vi "Call Fade-In Async.vi"(4 "Close on Fade-Out [T]":bool=TRUE, 5 "Delay (ms) [0]":i32, 6 "Fade Direction [Fade In]":enum16{"Fade In", "Fade Out"}(ring), 7 "Fade-In Time (ms)":u32=200, 8 "error in (no error)":errorcluster, 11 "Calling VI":refnum<vi>) -> (0 "error out":errorcluster)   [LabVIEW 2017]
doc: "Calls the Fade In/Out VI asynchronously so that other operations are not interrupted by this nicety.\n\nIf the calling VI Ref is not wired, the calling VIs parent is assumed, which is usally what you want."
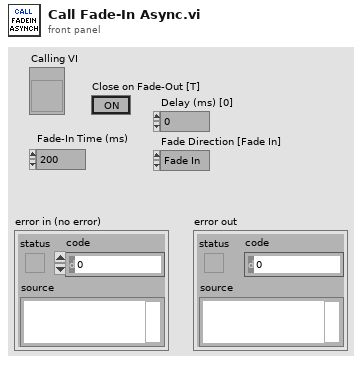
[diagram p1: front panel]
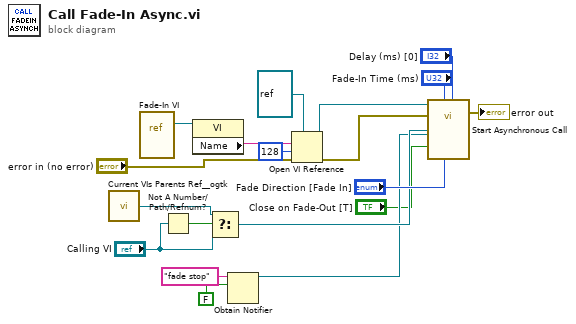
[diagram p0: block diagram]
diagram:
  n1 = call "Current VIs Parents Ref__ogtk.vi"() -> ("Calling VI's Reference"=w11:refnum<vi>)  [unwired: 2 in]
  n2 = vi-ref "Fade-In VI.vi"() -> (w16:refnum<vi>)
  n3 = Not A Number/Path/Refnum?(number/path/refnum="Calling VI") -> (NaN/Path/Refnum?=w12:bool)
  n4 = property class="VI"(reference=w16) -> ("Name"=w17:string)  [unwired: 1 in, 2 out]
  n5 = Select(t=w11, s=w12, f="Calling VI") -> (s? t:f=w9:refnum<vi>)
  n6 = Obtain Notifier(name (unnamed)="fade stop", notification data type=FALSE) -> (notifier out=w6:refnum<notifier>)  [unwired: 2 in, 2 out]
  n7 = Open VI Reference(type specifier VI Refnum (for type only)=refnum<vi> refnum, vi path=w17, options=128, error in (no error)="error in (no error)") -> (vi reference=w18:refnum<vi>, error out=w2:errorcluster)  [unwired: 2 in]
  n8 = call-by-ref "Start Asynchronous Call"(reference=w18, error in=w2, "Close on Fade-Out [T]"="Close on Fade-Out [T]", "Delay (ms) [0]"="Delay (ms) [0]", "Fade Direction [Fade In]"="Fade Direction [Fade In]", "Fade-in time (ms) [500]"="Fade-In Time (ms)", "stop notifier"=w6, "VI Ref"=w9) -> (error out=→"error out":errorcluster)  [unwired: 6 in, 1 out]
